vi "Read Iteration.vi"(8 "error in (no error)":errorcluster, 11 "Pixel in":refnum<class "Pixel.lvclass">) -> (0 "error out":errorcluster, 2 "Iteration":u16, 3 "Pixel out":refnum<class "Pixel.lvclass">)   [LabVIEW 2016, in "Pixel.lvclass"]
uses:
  Pixel.lvclass
  Pixel.lvclass/Pixel.ctl
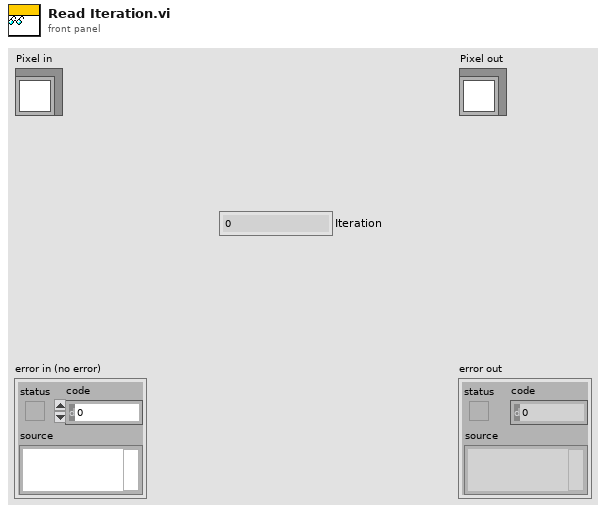
[diagram p1: front panel]
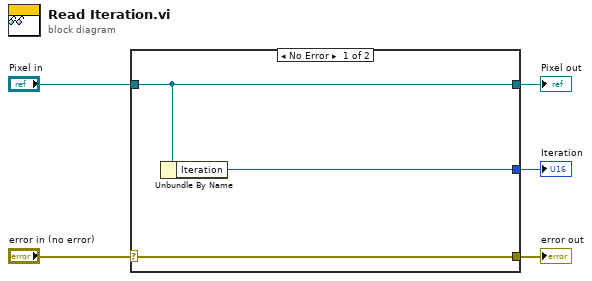
[diagram p0: block diagram]
diagram:
  n1 = case shown="No Error" "error in (no error)" {
    selector: "error in (no error)" -> [w8 w9]
    tunnel: [w8 w9] -> w4
    tunnel: [w7 w10] -> w2
    tunnel: "Pixel in" -> [w7 w10]
    tunnel: [w6 _] -> w1
    frame No Error {
      n2 = Unbundle By Name(w7) -> ("Iteration"=w6:u16)
    }
    frame Error {
    }
  }
  "error out" <- w4
  "Pixel out" <- w2
  "Iteration" <- w1
